vi "Snap Mark.vi"(11 "Main Page UIRef":T1) -> (0 "error out":errorcluster)   [LabVIEW 2019, in "MPC_Laser Marked.lvclass"]
uses:
  MPC_Laser Marked.lvclass
  Function/UpVision/Ctrl/UpColorImg.ctl
  Function/UpVision/Ctrl/UpEnum_VisionCalibSet_Act.ctl
  LLB/Message/MsgShowAndLog.lvlib
  Function/UpVision/Ctrl/UpGrayImg.ctl
  Function/IO Folder/IO_VI/IOCtrl/Ctrl/DMC1000B_1 SelectOutput.ctl
  Function/Main UI/Glb/Main_UI Gb.vi
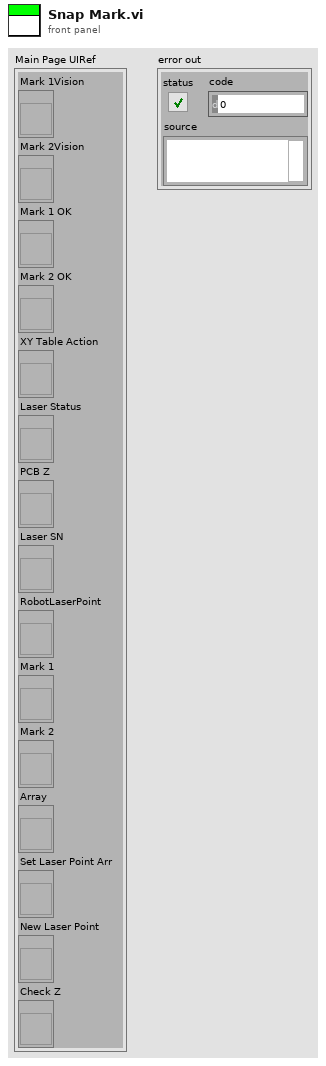
[diagram p1: front panel]
types:
  T1 = cluster{"Mark 1Vision":refnum<vi>, "Mark 2Vision":refnum<vi>, "Mark 1 OK":refnum<vi>, "Mark 2 OK":refnum<vi>, "XY Table Action":refnum<vi>, "Laser Status":refnum<vi>, "PCB Z":refnum<vi>, "Laser SN":refnum<vi>, "RobotLaserPoint":refnum<vi>, "Mark 1":refnum<vi>, "Mark 2":refnum<vi>, "Array":refnum<vi>, "Set Laser Point Arr":refnum<vi>, "New Laser Point":refnum<vi>, "Check Z":refnum<vi>}
  T2 = typedef "DMC1000B_1 SelectOutput.ctl" = enum16{"M_Out0預備", "M_OUT01蜂鳴器", "M_OUT02紅燈", "M_OUT03綠燈", "M_OUT04黃燈", "M_OUT05上頂固定位氣缸電磁閥", "M_OUT06到料阻擋氣缸電磁閥", "M_OUT07向前機台發出要料#1信號", "M_OUT08向前機台發出要料#2信號", "M_OUT09向後機台發出有料#3信號", "M_OUT10向後機台發出有料#4信號", "M_OUT11接駁台馬達啟動開/關", "M_OUT12接駁台馬達慢速", "M_OUT13抽風機開/關", "M_OUT14上視覺上光源", "M_OUT15DC吹風扇開/關", "M_OUT16Z軸煞車釋放", "M_OUT17", "M_OUT18", "M_OUT19", "M_OUT20", "M_OUT21", "M_OUT22", "M_OUT23", "M_OUT24", "M_OUT25第一軸SEVON1伺服使能信號", "M_OUT26第二軸SEVON2伺服使能信號", "M_OUT27第三軸SEVON3伺服使能信號"}
  T3 = typedef "UpEnum_VisionCalibSet_Act.ctl" = enum16{"initial", "initialref", "save", "load", "UpDataToUI", "write", "read"}
  T4 = typedef "UpColorImg.ctl" = enum16{"CUpCam", "CUpSource", "CUpShow", "CUpToProcess1", "CUpToProcess2", "CUpForMatch", "CUpForCheckNumbers", "CupPreProcess"}
  T5 = typedef "UpGrayImg.ctl" = enum16{"CUpGray", "CUpProce1", "CUpProce2", "UpPattern1", "UpPattern2", "UpCalibImg", "UpPreProcess"}
  T6 = typedef "IMAQ Image.ctl" = refnum<image>
  T7 = cluster{"Position":cluster{"x":sgl, "y":sgl}, "Angle":sgl, "Score":sgl}
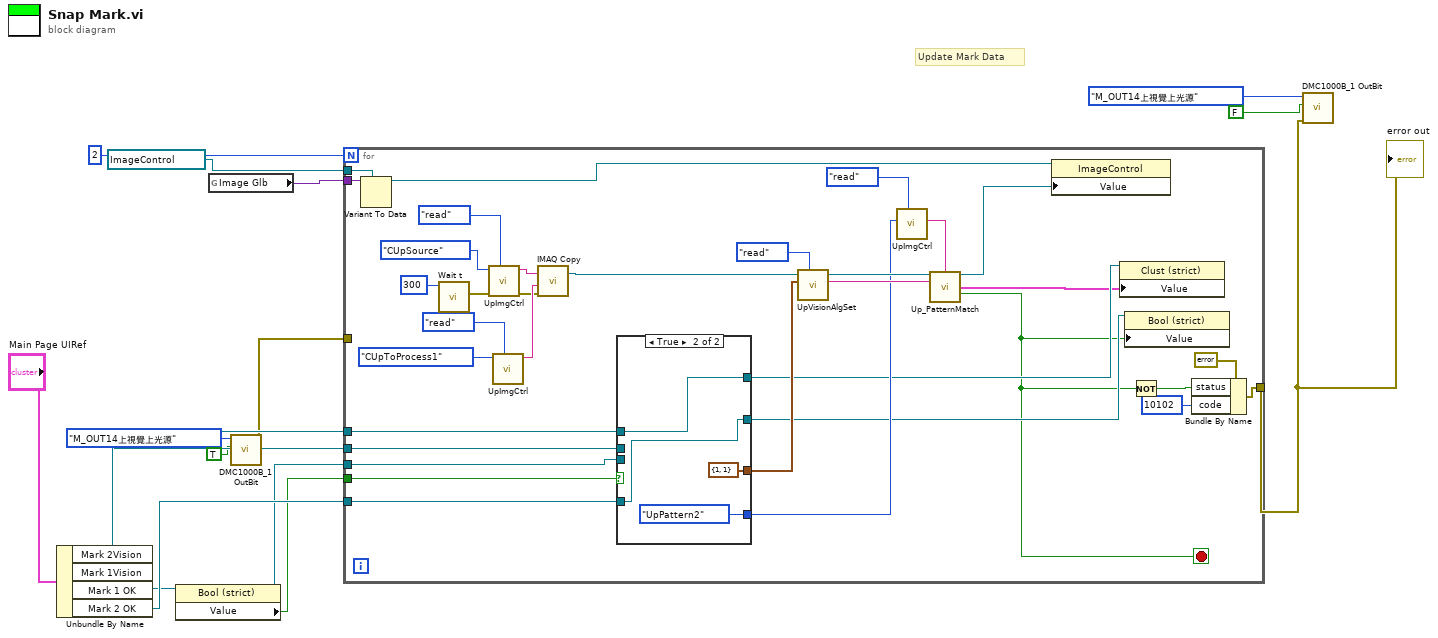
[diagram p0: block diagram]
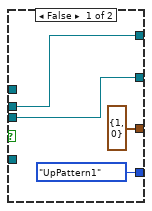
[diagram p2: hidden frame]
diagram:
  # "Update Mark Data"
  n1 = Unbundle By Name("Main Page UIRef") -> ("Mark 2Vision"=w12:refnum<vi>, "Mark 1Vision"=w11:refnum<vi>, "Mark 1 OK"=w8:refnum<vi>, "Mark 2 OK"=w14:refnum<vi>)
  n2 = property class="Bool (strict)"(reference=w8) -> (reference out=w13:refnum<vi>, "Value"=w10:bool)  [unwired: 1 in, 1 out]
  n3 = global read "Main_UI Gb.vi" "Image Glb"() -> (w15:variant)
  n4 = call "DMC1000B_1 OutBit.vi"("BL"=TRUE, "IO_Output_1 Select"=DMC1000B_1_SelectOutput."M_OUT14上視覺上光源") -> ("error out"=w4:errorcluster)  [unwired: 9 in]
  n5 = for {
    N: 2 -> [_]
    tunnel: [w33] -> w7
    tunnel: w4 -> [_]
    tunnel: w10 -> [w28]
    tunnel: w11 -> [w27]
    tunnel: w12 -> [w26]
    tunnel: w13 -> [w23]
    tunnel: w14 -> [w20]
    tunnel: w15 -> [w19]
    tunnel: refnum<vi> refnum ("Image") -> [w18]
    stop <- w21 stop-if-true
    n6 = Variant To Data(type=w18, Variant=w19) -> (data=w17:refnum<vi>)  [unwired: 1 in, 1 out]
    n7 = call "Wait t.vi"("wait(ms)"=u32 300) -> ("error out"=w42:errorcluster)  [unwired: 10 in]
    n8 = call "UpImgCtrl.vi"("Action"=enum16{"Initial", "read", "release"}."read", "error in (no error)"=w42, "ColorImg 2"=UpColorImg."CUpSource") -> ("error out"=w41:errorcluster, "ColorImg"=w44:string)  [unwired: 6 in, 1 out]
    n9 = call "UpImgCtrl.vi"("Action"=enum16{"Initial", "read", "release"}."read", "ColorImg 2"=UpColorImg."CUpToProcess1") -> ("ColorImg"=w43:string)  [unwired: 7 in, 2 out]
    n10 = call "IMAQ Copy"("error in (no error)"=w41, "Image Dst"=w43, "Image Src"=w44) -> ("Image Dst Out"=w40:T6)  [unwired: 3 in, 1 out]
    n11 = case shown="True" w28 {
      tunnel: [cluster{"Y":i32, "X":i32} {"Y"=1, "X"=0} ("indedx") cluster{"Y":i32, "X":i32} {"Y"=1, "X"=1} ("indedx")] -> w38
      tunnel: [UpGrayImg."UpPattern1" ("GrayImg 2") UpGrayImg."UpPattern2" ("GrayImg 2")] -> w35
      tunnel: w27 -> [w50 _]
      tunnel: [w50 w55] -> w25
      tunnel: w26 -> [_ w55]
      tunnel: w23 -> [w51 _]
      tunnel: [w51 w54] -> w22
      tunnel: w20 -> [_ w54]
      frame False {
      }
      frame True {
      }
    }
    n12 = call "UpVisionAlgSet.vi"("Enum"=UpEnum_VisionCalibSet_Act."read", "indedx"=w38) -> ("DataOut"=w37:string)  [unwired: 7 in, 2 out]
    n13 = call "UpImgCtrl.vi"("Action"=enum16{"Initial", "read", "release"}."read", "GrayImg 2"=w35) -> ("GrayImg"=w34:string)  [unwired: 7 in, 2 out]
    n14 = call "Up_PatternMatch.vi"("Image In"=w40, "Template Image"=w34, "ROIIn"=w37) -> ("Image Out"=w29:T6, "ResultShow"=w24:T7, "OK"=w21:bool)  [unwired: 6 in, 4 out]
    n15 = property class="ImageControl"(reference=w17, "Value"=w29) -> ()  [unwired: 1 in, 2 out]
    n16 = property class="Clust (strict)"(reference=w25, "Value"=w24) -> ()  [unwired: 1 in, 2 out]
    n17 = property class="Bool (strict)"(reference=w22, "Value"=w21) -> ()  [unwired: 1 in, 2 out]
    n18 = Not(x=w21) -> (.not. x?=w31:bool)
    n19 = Bundle By Name(cluster=errorcluster {"status"=FALSE, "code"=0, "source"=""} ("error constant"), "status"=w31, "code"=10102) -> (w33:errorcluster)
  }
  "error out" <- w7
  n20 = call "DMC1000B_1 OutBit.vi"("error in (no error)"=w7, "BL"=FALSE, "IO_Output_1 Select"=DMC1000B_1_SelectOutput."M_OUT14上視覺上光源") -> ()  [unwired: 8 in, 1 out]
